vi "JSON read.vi"(8 "error in (no error)":errorcluster, 11 "ZenGage v3.0 UI in":T1) -> (0 "error out":errorcluster, 3 "ZenGage v3.0 UI in":T1)   [LabVIEW 2019, in "ZenGage v3.0 UI.lvclass"]
uses:
  ZenGage v3.0 UI.lvclass
  <vilib>/Utility/miscctls.llb/LVRowAndColumnTypeDef.ctl
  Type Definitions/Controls and Indicators/Select a part (combobox).ctl
  Type Definitions/Controls and Indicators/EDL control references.ctl
  Type Definitions/Controls and Indicators/Diagnostics control referencs.ctl
  Type Definitions/Controls and Indicators/Inspection control references.ctl
  Type Definitions/Controls and Indicators/General_Control references.ctl
  Type Definitions/Controls and Indicators/Controls and Indicators Cluster.ctl
  Type Definitions/JSON Read/UI JSON read cluster.ctl
  Type Definitions/General/JSONRead.ctl
  Type Definitions/Inspection/Inspection Cluster.ctl
  Type Definitions/Diagnostics/Diagnostics(Cluster).ctl
  Type Definitions/Edit tolerance settings/Rack Selection.ctl
  <vilib>/Utility/miscctls.llb/LVPoint32TypeDef.ctl
  Type Definitions/Edit tolerance settings/Edit Tolerance Input.ctl
  Type Definitions/Edit tolerance settings/Edit Tolerance Overall Cluster.ctl
  Common/Controls/Pop-up Input.ctl
  Type Definitions/General/UI States(UI button enable disable).ctl
  Type Definitions/General/UIDataCluster.ctl
  Type Definitions/General/Master sample references.ctl
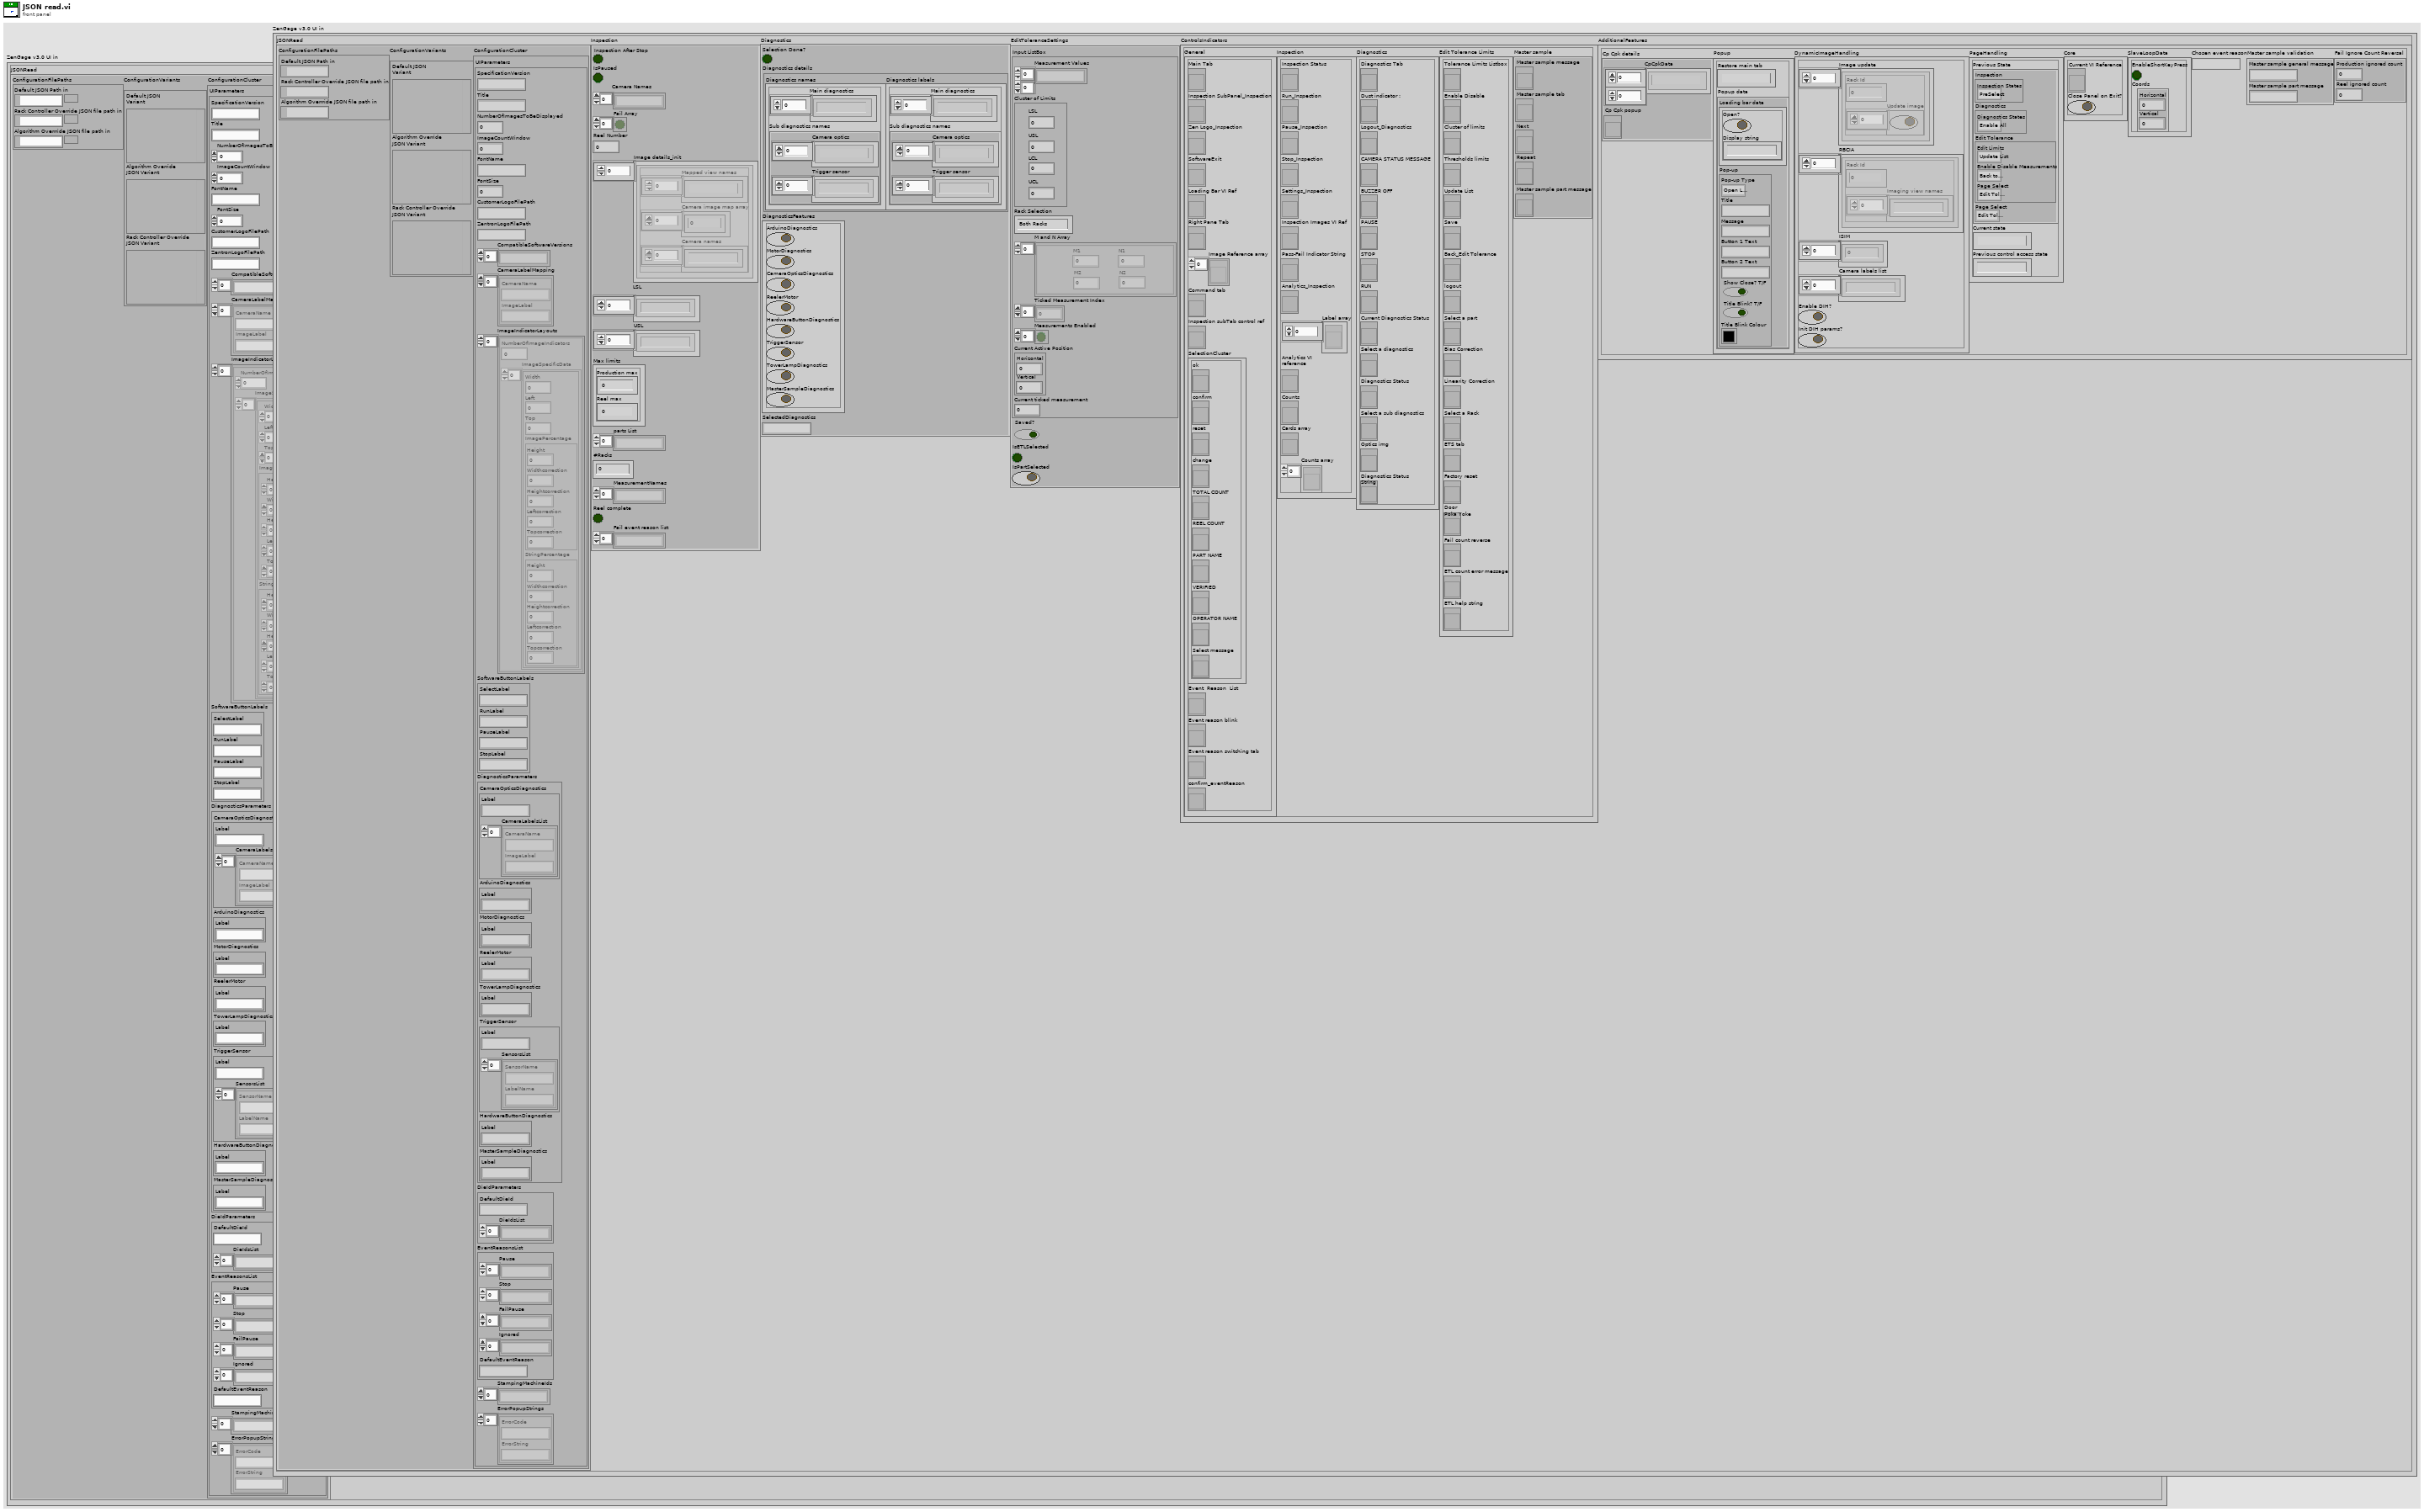
[diagram p1: front panel]
types:
  T1 = typedef "UIDataCluster.ctl" = cluster{"JSONRead":T2, "Inspection":T4, "Diagnostics":T5, "EditToleranceSettings":T6, "ControlsIndicators":T10, "AdditionalFeatures":cluster{"Cp Cpk details":cluster{"CpCpkData":string[][], "Cp Cpk popup":refnum<vi>}, "Popup":cluster{"Restore main tab":string, "Popup data":cluster{"Loading bar data":cluster{"Open?":bool, "Display string":string}, "Pop-up":T16}}, "DynamicImageHandling":cluster{"Image update":cluster{"Rack Id":i32, "Update image":bool[]}[], "RBCIA":cluster{"Rack Id":u8, "Imaging view names":string[]}[], "ISIM":u8[], "Camera labels list":string[], "Enable DIH?":bool, "Init DIH params?":bool}, "PageHandling":cluster{"Previous State":T17, "Current state":string, "Previous control access state":string}, "Core":cluster{"Current VI Reference":refnum<vi>, "Close Panel on Exit?":bool}, "SlaveLoopData":cluster{"EnableShortKeyPress":bool, "Point32":T9}, "Chosen event reason":string, "Master sample validation":cluster{"Master sample general message":string, "Master sample part message":string}, "Fail Ignore Count Reversal":cluster{"Production ignored count":u64, "Reel ignored count":u64}}}
  T2 = typedef "ZenGage v3.0 UI.lvclass/JSONRead.ctl" = cluster{"ConfigurationFilePaths":cluster{"Default JSON Path in":path, "Rack Controller Override JSON file path in":path, "Algorithm Overrride JSON file path in ":path}, "ConfigurationVariants":cluster{"Default JSON \nVariant":variant, "Algorithm Override\nJSON Variant":variant, "Rack Controller Override\nJSON Variant":variant}, "ConfigurationCluster":T3}
  T3 = typedef "ZenGage v3.0 UI.lvclass/UI JSON read cluster.ctl" = cluster{"UIParameters":cluster{"SpecificationVersion":string, "Title":string, "NumberOfImagesToBeDisplayed":dbl, "ImageCountWindow":dbl, "FontName":string, "FontSize":dbl, "CustomerLogoFilePath":string, "ZentronLogoFilePath":string, "CompatibleSoftwareVersions":string[], "CameraLabelMapping":cluster{"CameraName":string, "ImageLabel":string}[], "ImageIndicatorLayouts":cluster{"NumberOfImageIndicators":dbl, "ImageSpecificData":cluster{"Width":dbl, "Left":dbl, "Top":dbl, "ImagePercentage":cluster{"Height":dbl, "Widthcorrection":i64, "Heightcorrection":i64, "Leftcorrection":dbl, "Topcorrection":dbl}, "StringPercentage":cluster{"Height":dbl, "Widthcorrection":i64, "Heightcorrection":dbl, "Leftcorrection":dbl, "Topcorrection":dbl}}[]}[], "SoftwareButtonLabels":cluster{"SelectLabel":string, "RunLabel":string, "PauseLabel":string, "StopLabel":string}, "DiagnosticsParameters":cluster{"CameraOpticsDiagnostics":cluster{"Label":string, "CameraLabelsList":cluster{"CameraName":string, "ImageLabel":string}[]}, "ArduinoDiagnostics":cluster{"Label":string}, "MotorDiagnostics":cluster{"Label":string}, "ReelerMotor":cluster{"Label":string}, "TowerLampDiagnostics":cluster{"Label":string}, "TriggerSensor":cluster{"Label":string, "SensorsList":cluster{"SensorName":string, "LabelName":string}[]}, "HardwareButtonDiagnostics":cluster{"Label":string}, "MasterSampleDiagnostics":cluster{"Label":string}}, "DieIdParameters":cluster{"DefaultDieId":string, "DieIdsList":string[]}, "EventReasonsList":cluster{"Pause":string[], "Stop":string[], "FailPause":string[], "Ignored":string[], "DefaultEventReason":string}, "StampingMachineIds":string[], "ErrorPopupStrings":cluster{"ErrorCode":string, "ErrorString":string}[]}}
  T4 = typedef "ZenGage v3.0 UI.lvclass/Inspection Cluster.ctl" = cluster{"Inspection After Stop":bool, "IsPaused":bool, "Camera Names":string[], "Fail Array":bool[], "Reel Number":u32, "Image details_init":cluster{"Mapped view names":string[], "Camera image map array":i32[], "Camera names":string[]}[], "LSL":string[], "USL":string[], "Max limits":cluster{"Production max":u64, "Reel max":u64}, "parts List":string[], "#Racks":u8, "MeasurementNames":string[], "Reel complete":bool, "Fail event reason list":string[]}
  T5 = typedef "ZenGage v3.0 UI.lvclass/Diagnostics(Cluster).ctl" = cluster{"Selection Done?":bool, "Diagnostics details":cluster{"Diagnostics names":cluster{"Main diagnostics":string[], "Sub diagnostics names":cluster{"Camera optics":string[], "Trigger sensor":string[]}}, "Diagnostics labels":cluster{"Main diagnostics":string[], "Sub diagnostics names":cluster{"Camera optics":string[], "Trigger sensor":string[]}}}, "DiagnosticsFeatures":cluster{"ArduinoDiagnostics":bool, "MotorDiagnostics":bool, "CameraOpticsDiagnostics":bool, "ReelerMotor":bool, "HardwareButtonDiagnostics":bool, "TriggerSensor":bool, "TowerLampDiagnostics":bool, "MasterSampleDiagnostics":bool}, "SelectedDiagnostics":string}
  T6 = typedef "ZenGage v3.0 UI.lvclass/Edit Tolerance Overall Cluster.ctl" = cluster{"Input ListBox":T7, "Saved?":bool, "IsETLSelected":bool, "IsPartSelected":bool}
  T7 = typedef "ZenGage v3.0 UI.lvclass/Edit Tolerance Input.ctl" = cluster{"Measurement Values":string[][], "Cluster of Limits":cluster{"LSL":dbl, "USL":dbl, "LCL":dbl, "UCL":dbl}, "Rack Selection":T8, "M and N Array":cluster{"M1":u64, "M2":u64, "N1":u64, "N2":u64}[], "Ticked Measurement Index":u32[], "Measurements Enabled":bool[], "Current Active Position":T9, "Current ticked measurement":dbl}
  T8 = typedef "ZenGage v3.0 UI.lvclass/Rack Selection.ctl" = enum16{"Both Racks", "Rack 2", "Rack 1"}
  T9 = typedef "LVPoint32TypeDef.ctl" = cluster{"Horizontal":i32, "Vertical":i32}
  T10 = typedef "ZenGage v3.0 UI.lvclass/Controls and Indicators Cluster.ctl" = cluster{"General":T11, "Inspection":T12, "Diagnostics":T13, "Edit Tolerance Limits":T14, "Master sample":T15}
  T11 = typedef "ZenGage v3.0 UI.lvclass/General_Control references.ctl" = cluster{"Main Tab":refnum<vi>, "Inspection SubPanel_Inspection":refnum<vi>, "Zen Logo_Inspection":refnum<vi>, "SoftwareExit":refnum<vi>, "Loading Bar VI Ref":refnum<vi>, "Right Pane Tab":refnum<vi>, "Image Reference array":refnum<vi>[], "Command tab":refnum<vi>, "Inspection subTab control ref":refnum<vi>, "SelectionCluster":cluster{"ok":refnum<vi>, "confirm":refnum<vi>, "reset":refnum<vi>, "change":refnum<vi>, "TOTAL COUNT":refnum<vi>, "REEL COUNT":refnum<vi>, "PART NAME":refnum<vi>, "VERIFIED":refnum<vi>, "OPERATOR NAME":refnum<vi>, "Select message":refnum<vi>}, "Event  Reason  List":refnum<vi>, "Event reason blink":refnum<vi>, "Event reason switching tab":refnum<vi>, "confirm_eventReason":refnum<vi>}
  T12 = typedef "ZenGage v3.0 UI.lvclass/Inspection control references.ctl" = cluster{"Inspection Status":refnum<vi>, "Run_Inspection":refnum<vi>, "Pause_Inspection":refnum<vi>, "Stop_Inspection":refnum<vi>, "Settings_Inspection":refnum<vi>, "Inspection Images VI Ref":refnum<vi>, "Pass-Fail Indicator String":refnum<vi>, "Analytics_Inspection":refnum<vi>, "Label array":refnum<vi>[], "Analytics VI\nreference":refnum<vi>, "Counts":refnum<vi>, "Cards array":refnum<vi>, "Counts array":refnum<vi>[]}
  T13 = typedef "ZenGage v3.0 UI.lvclass/Diagnostics control referencs.ctl" = cluster{"Diagnostics Tab":refnum<vi>, "Dust indicator :":refnum<vi>, "Logout_Diagnostics":refnum<vi>, "CAMERA STATUS MESSAGE":refnum<vi>, "BUZZER OFF":refnum<vi>, "PAUSE":refnum<vi>, "STOP":refnum<vi>, "RUN":refnum<vi>, "Current Diagnostics Status":refnum<vi>, "Select a diagnostics":refnum<vi>, "Diagnostics Status":refnum<vi>, "Select a sub diagnostics":refnum<vi>, "Optics img":refnum<vi>, "Diagnostics Status\nString":refnum<vi>}
  T14 = typedef "ZenGage v3.0 UI.lvclass/EDL control references.ctl" = cluster{"Tolerance Limits Listbox":refnum<vi>, "Enable Disable":refnum<vi>, "Cluster of limits":refnum<vi>, "Thresholds limits":refnum<vi>, "Update List":refnum<vi>, "Save":refnum<vi>, "Back_Edit Tolerance":refnum<vi>, "logout":refnum<vi>, "Select a part":refnum<vi>, "Bias Correction":refnum<vi>, "Linearity Correction":refnum<vi>, "Select a Rack":refnum<vi>, "ETS tab":refnum<vi>, "Factory reset":refnum<vi>, "Door\nPoka Yoke":refnum<vi>, "Fail count reverse":refnum<vi>, "ETL count error message":refnum<vi>, "ETL help string":refnum<vi>}
  T15 = typedef "Master sample references.ctl" = cluster{"Master sample message":refnum<vi>, "Master sample tab":refnum<vi>, "Next":refnum<vi>, "Repeat":refnum<vi>, "Master sample part message":refnum<vi>}
  T16 = typedef "Pop-up Input.ctl" = cluster{"Pop-up Type":enum16{"Open Logo Display", "Close Logo Display", "Open Loading Bar", "Close Loading Bar", "Open Alert Display", "Close Alert Display", "One button dialog box", "Two button dialog box", "User Authentication"}, "Title":string, "Message":string, "Button 1 Text":string, "Button 2 Text":string, "Show Close? T/F":bool, "Title Blink? T/F":bool, "Title Blink Colour":u32}
  T17 = typedef "ZenGage v3.0 UI.lvclass/UI States(UI button enable disable).ctl" = cluster{"Inspection":cluster{"Inspection States":enum16{"PreSelect", "Back _Inspection", "Analytics", "Ready To Run", "Ready To Insert", "Enable All buttons", "Disable All Buttons", "Settings", "Select", "Stop", "Pause", "Inspect"}}, "Diagnostics":cluster{"Diagnostics States":enum16{"Enable All", "Camera Optics Fail", "Loading Bar", "Camera Optics", "Motor", "Arduino", "POST Done", "POST"}}, "Edit Tolerance":cluster{"Edit Limits":enum16{"Update List"}, "Enable Disable Measurements":enum16{"Back to Edit Tolerance"}, "Page Select":enum16{"Edit Tolerance Limits", "Enable Disable Buttons"}}, "Page Select":enum16{"Edit Tolerance", "Diagnostics", "Inspection"}}
  T18 = enum32{"Edit Tolerance Limits1", "Inspection", "Master sample", "Diagnostics"}
  T19 = enum8{"Enabled", "Disabled", "Disabled and Grayed Out"}
  T20 = enum32{"Analytics", "Blank", "Diagnostics", "Run", "Edit Tolerance Settings"}
  T21 = typedef "LVRowAndColumnTypeDef.ctl" = cluster{"Row":i32, "Column":i32}
  T22 = cluster{"CameraOpticsDiagnostics":cluster{"Label":string, "CameraLabelsList":cluster{"CameraName":string, "ImageLabel":string}[]}, "ArduinoDiagnostics":cluster{"Label":string}, "MotorDiagnostics":cluster{"Label":string}, "ReelerMotor":cluster{"Label":string}, "TowerLampDiagnostics":cluster{"Label":string}, "TriggerSensor":cluster{"Label":string, "SensorsList":cluster{"SensorName":string, "LabelName":string}[]}, "HardwareButtonDiagnostics":cluster{"Label":string}, "MasterSampleDiagnostics":cluster{"Label":string}}
  T23 = cluster{"Diagnostics names":cluster{"Main diagnostics":string[], "Sub diagnostics names":cluster{"Camera optics":string[], "Trigger sensor":string[]}}, "Diagnostics labels":cluster{"Main diagnostics":string[], "Sub diagnostics names":cluster{"Camera optics":string[], "Trigger sensor":string[]}}}
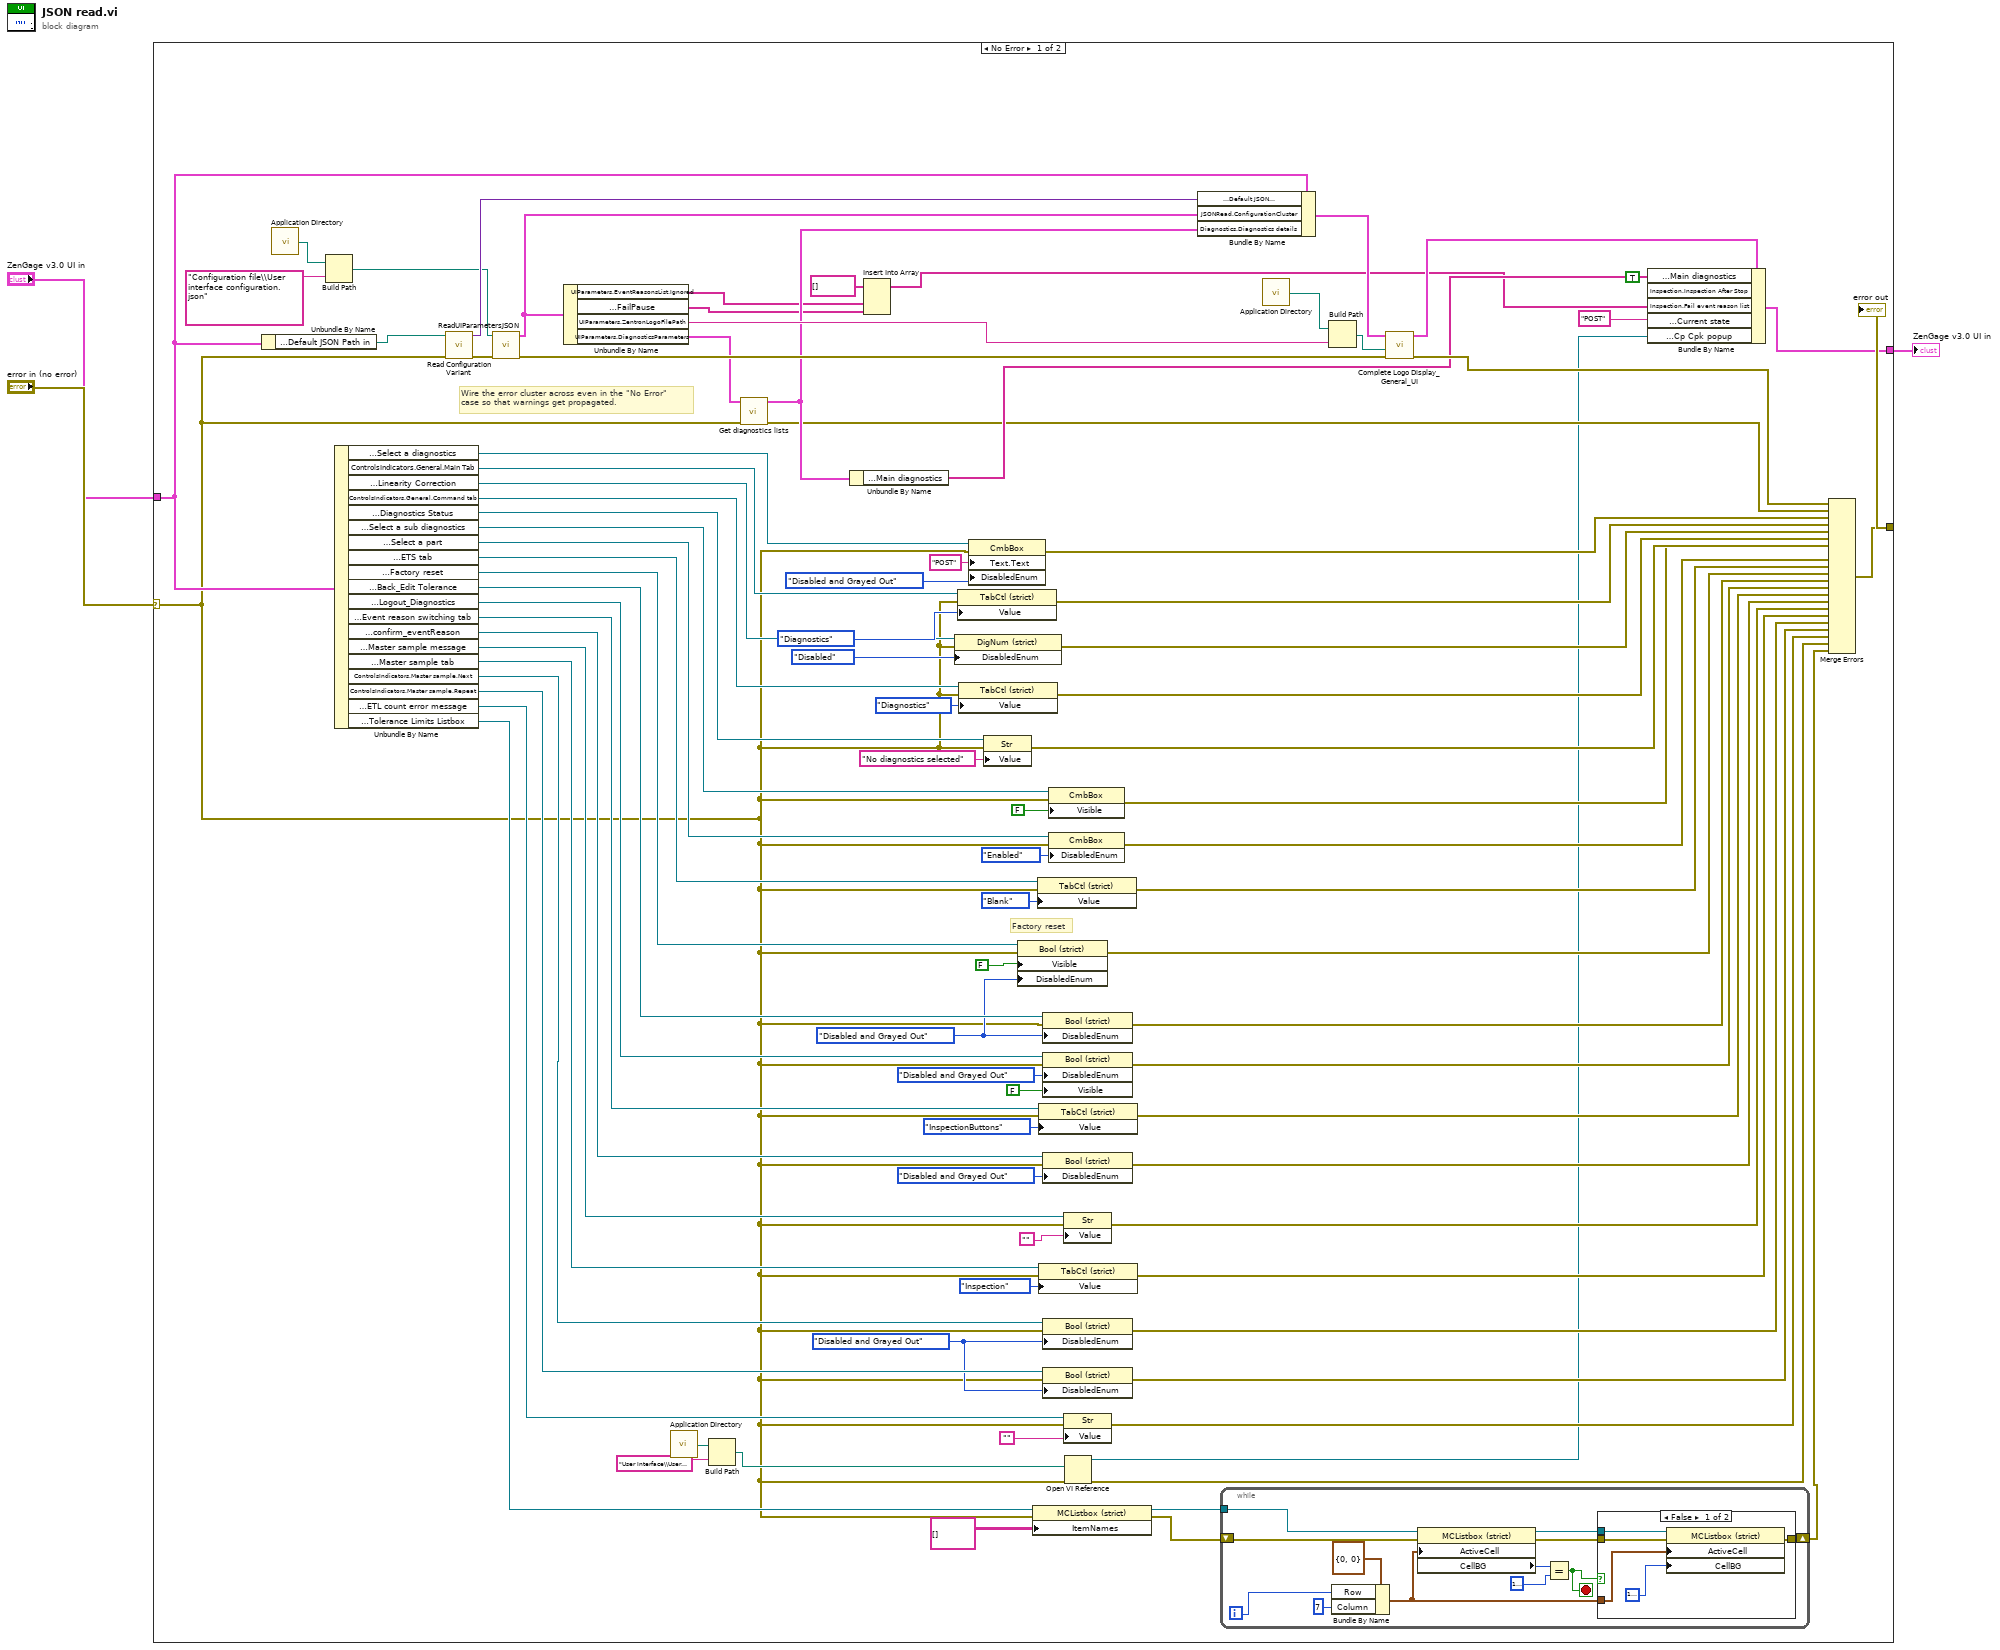
[diagram p0: block diagram]
diagram:
  n1 = case shown="No Error" "error in (no error)" {
    selector: "error in (no error)" -> [w9 w117]
    tunnel: [w89 w117] -> w3
    tunnel: [w82 w116] -> w1
    tunnel: "ZenGage v3.0 UI in" -> [w59 w116]
    frame No Error {
      w29 = T19."Disabled and Grayed Out" ("Disabled")
      w48 = T19."Disabled and Grayed Out" ("Disabled")
      # "Factory reset"
      # "Wire the error cluster across even in the \"No Error\"\ncase so that warnings get propagated."
      n2 = Unbundle By Name(w59) -> ("JSONRead.ConfigurationFilePaths.Default JSON Path in"=w97:path)
      n3 = call <vilib>:"Application Directory.vi"() -> ("Application Directory"=w76:path)
      n4 = Build Path(base path=w76, name or relative path="Configuration file\\User interface configuration.json") -> (appended path=w74:path)
      n5 = Unbundle By Name(w59) -> ("ControlsIndicators.Diagnostics.Select a diagnostics"=w52:refnum<vi>, "ControlsIndicators.General.Main Tab"=w88:refnum<vi>, "ControlsIndicators.Edit Tolerance Limits.Linearity Correction"=w85:refnum<vi>, "ControlsIndicators.General.Command tab"=w81:refnum<vi>, "ControlsIndicators.Diagnostics.Diagnostics Status"=w79:refnum<vi>, "ControlsIndicators.Diagnostics.Select a sub diagnostics"=w72:refnum<vi>, "ControlsIndicators.Edit Tolerance Limits.Select a part"=w69:refnum<vi>, "ControlsIndicators.Edit Tolerance Limits.ETS tab"=w56:refnum<vi>, "ControlsIndicators.Edit Tolerance Limits.Factory reset"=w53:refnum<vi>, "ControlsIndicators.Edit Tolerance Limits.Back_Edit Tolerance"=w61:refnum<vi>, "ControlsIndicators.Diagnostics.Logout_Diagnostics"=w49:refnum<vi>, "ControlsIndicators.General.Event reason switching tab"=w45:refnum<vi>, "ControlsIndicators.General.confirm_eventReason"=w38:refnum<vi>, "ControlsIndicators.Master sample.Master sample message"=w37:refnum<vi>, "ControlsIndicators.Master sample.Master sample tab"=w36:refnum<vi>, "ControlsIndicators.Master sample.Next"=w35:refnum<vi>, "ControlsIndicators.Master sample.Repeat"=w34:refnum<vi>, "ControlsIndicators.Edit Tolerance Limits.ETL count error message"=w25:refnum<vi>, "ControlsIndicators.Edit Tolerance Limits.Tolerance Limits Listbox"=w10:refnum<vi>)
      n6 = call "Read Configuration Variant.vi"("error in"=w9, "JSON file path in"=w97) -> ("error out"=w96:errorcluster, "JSON variant out"=w92:variant)  [unwired: 8 in]
      n7 = call "ReadUIParametersJSON.vi"("error in"=w96, "User interface JSON filepath"=w74) -> ("error out"=w91:errorcluster, "UI JSON"=w73:T3)  [unwired: 8 in]
      n8 = Unbundle By Name(w73) -> ("UIParameters.EventReasonsList.Ignored"=w21:string[], "UIParameters.EventReasonsList.FailPause"=w20:string[], "UIParameters.ZentronLogoFilePath"=w93:string, "UIParameters.DiagnosticsParameters"=w22:T22)
      n9 = call <vilib>:"Application Directory.vi"() -> ("Application Directory"=w15:path)
      n10 = Build Path(base path=w15, name or relative path="User Interface\\User Interface Actor\\SubVIs\\Inspection\\Inspection\\Cp-Cpk Popup.vi") -> (appended path=w14:path)
      n11 = call "Get diagnostics lists.vi"("error in (no error)"=w9, "UIParameters.DiagnosticsParameters"=w22) -> ("error out"=w57:errorcluster, "Diagnostics details"=w64:T23)  [unwired: 8 in]
      n12 = Unbundle By Name(w64) -> ("Diagnostics labels.Main diagnostics"=w65:string[])
      n13 = Insert Into Array(array=string[] [], new element #1=w21, new element #2=w20) -> (w18:string[])  [unwired: 1 in]
      n14 = property class="DigNum (strict)"(reference=w85, error in=w9, "DisabledEnum"=T19."Disabled" ("Disabled")) -> (error out=w83:errorcluster)  [unwired: 1 out]
      n15 = property class="TabCtl (strict)"(reference=w88, error in=w9, "Value"=T20."Diagnostics") -> (error out=w86:errorcluster)  [unwired: 1 out]
      n16 = property class="TabCtl (strict)"(reference=w81, error in=w9, "Value"=T18."Diagnostics") -> (error out=w80:errorcluster)  [unwired: 1 out]
      n17 = property class="CmbBox"(reference=w52, error in=w9, "Text.Text"="POST", "DisabledEnum"=T19."Disabled and Grayed Out" ("Disabled")) -> (error out=w50:errorcluster)  [unwired: 1 out]
      n18 = property class="Str"(reference=w79, error in=w9, "Value"="No diagnostics selected") -> (error out=w77:errorcluster)  [unwired: 1 out]
      n19 = property class="Bool (strict)"(reference=w53, error in=w9, "Visible"=FALSE, "DisabledEnum"=w48) -> (error out=w54:errorcluster)  [unwired: 1 out]
      n20 = property class="MCListbox (strict)"(reference=w10, error in=w9, "ItemNames"=string[][] [] ("Item Names")) -> (reference out=w7:refnum<vi>, error out=w6:errorcluster)
      n21 = property class="TabCtl (strict)"(reference=w56, error in=w9, "Value"=enum32{"Display", "Blank"}."Blank") -> (error out=w62:errorcluster)  [unwired: 1 out]
      n22 = property class="TabCtl (strict)"(reference=w45, error in=w9, "Value"=enum32{"EventReason", "InspectionButtons"}."InspectionButtons") -> (error out=w43:errorcluster)  [unwired: 1 out]
      n23 = property class="TabCtl (strict)"(reference=w36, error in=w9, "Value"=enum32{"Master sample", "Inspection"}."Inspection") -> (error out=w32:errorcluster)  [unwired: 1 out]
      n24 = property class="Bool (strict)"(reference=w61, error in=w9, "DisabledEnum"=w48) -> (error out=w60:errorcluster)  [unwired: 1 out]
      n25 = property class="Bool (strict)"(reference=w49, error in=w9, "DisabledEnum"=T19."Disabled and Grayed Out" ("Disabled"), "Visible"=FALSE) -> (error out=w47:errorcluster)  [unwired: 1 out]
      n26 = property class="Bool (strict)"(reference=w38, error in=w9, "DisabledEnum"=T19."Disabled and Grayed Out" ("Disabled")) -> (error out=w40:errorcluster)  [unwired: 1 out]
      n27 = property class="Bool (strict)"(reference=w35, error in=w9, "DisabledEnum"=w29) -> (error out=w31:errorcluster)  [unwired: 1 out]
      n28 = property class="Bool (strict)"(reference=w34, error in=w9, "DisabledEnum"=w29) -> (error out=w30:errorcluster)  [unwired: 1 out]
      n29 = property class="CmbBox"(reference=w72, error in=w9, "Visible"=FALSE) -> (error out=w71:errorcluster)  [unwired: 1 out]
      n30 = property class="CmbBox"(reference=w69, error in=w9, "DisabledEnum"=T19."Enabled" ("Disabled")) -> (error out=w67:errorcluster)  [unwired: 1 out]
      n31 = property class="Str"(reference=w37, error in=w9, "Value"="") -> (error out=w33:errorcluster)  [unwired: 1 out]
      n32 = property class="Str"(reference=w25, error in=w9, "Value"="") -> (error out=w23:errorcluster)  [unwired: 1 out]
      n33 = Open VI Reference(vi path=w14, error in (no error)=w9) -> (vi reference=w11:refnum<vi>, error out=w12:errorcluster)  [unwired: 4 in]
      n34 = Bundle By Name(cluster=w59, "JSONRead.ConfigurationVariants.Default JSON \nVariant"=w92, "JSONRead.ConfigurationCluster"=w73, "Diagnostics.Diagnostics details"=w64) -> (w58:T1)
      n35 = while {
        tunnel: w7 -> [w109]
        shift-right: [w102] -> w5
        shift-left: w6 -> [w108]
        i -> [w106]
        stop <- w98 stop-if-true
        n36 = Bundle By Name(cluster=T21 {"Row"=0, "Column"=0} ("Active Cell:Active Cell"), "Row"=w106, "Column"=7) -> (w100:T21)
        n37 = property class="MCListbox (strict)"(reference=w109, error in=w108, "ActiveCell"=w100) -> (reference out=w101:refnum<vi>, error out=w103:errorcluster, "CellBG"=w104:u32)
        n38 = Equal?(x=w104, y=u32 16777216) -> (x = y?=w98:bool)
        n39 = case shown="False" w98 {
          tunnel: w103 -> [w114 w115]
          tunnel: [w113 w115] -> w102
          tunnel: w101 -> [w112 _]
          tunnel: w100 -> [w110 _]
          frame False {
            n40 = property class="MCListbox (strict)"(reference=w112, error in=w114, "ActiveCell"=w110, "CellBG"=u32 16777216) -> (error out=w113:errorcluster)  [unwired: 1 out]
          }
          frame True {
          }
        }
      }
      n41 = call <vilib>:"Application Directory.vi"() -> ("Application Directory"=w95:path)
      n42 = Build Path(base path=w95, name or relative path=w93) -> (appended path=w94:path)
      n43 = call "Complete Logo Display_General_UI.vi"("error in (no error)"=w91, "ZenLogo file path in"=w94, "Cluster in"=w58) -> ("error out"=w66:errorcluster, "Cluster in"=w90:T1)  [unwired: 7 in]
      n44 = Bundle By Name(cluster=w90, "Diagnostics.Diagnostics details.Diagnostics labels.Main diagnostics"=w65, "Inspection.Inspection After Stop"=TRUE, "Inspection.Fail event reason list"=w18, "AdditionalFeatures.PageHandling.Current state"="POST", "AdditionalFeatures.Cp Cpk details.Cp Cpk popup"=w11) -> (w82:T1)
      n45 = Merge Errors(w66, w57, w50, w86, w83, w80, w77, w71, w67, w62, w54, w60, w47, w43, w40, w33, w32, w31, w30, w23, w12, w5) -> (w89:errorcluster)
    }
    frame Error {
    }
  }
  "error out" <- w3
  "ZenGage v3.0 UI in" <- w1
